vi "Write Packet.vi"(8 "error in (no error)":errorcluster, 9 "SessionMailbox in":refnum<queue>, 10 "Outgoing":T1, 11 "MQTT_Base in":refnum<class "MQTT_Base.lvclass">) -> (0 "error out":errorcluster, 3 "MQTT_Base out":refnum<class "MQTT_Base.lvclass">)   [LabVIEW 2013, in "MQTT Base.lvlib" / "MQTT_Base.lvclass"]
uses:
  MQTT_Base.lvclass
  Response -- cluster.ctl
  <vilib>/LabVIEW Open Source Project/MQTT Control Packets/Control Packets/ControlPacket/ControlPacket.lvclass
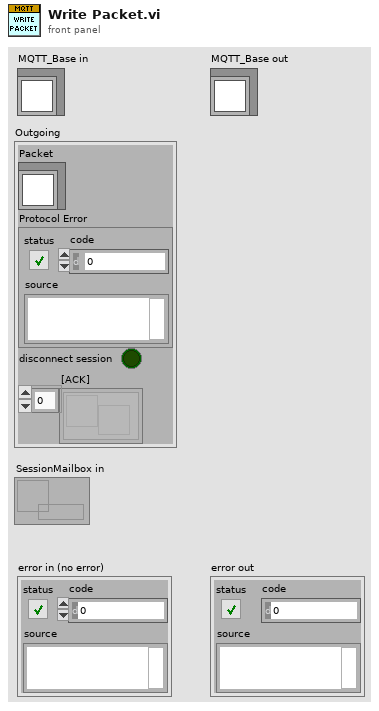
[diagram p1: front panel]
types:
  T1 = typedef "MQTT Base.lvlib/MQTT_Base.lvclass/Response -- cluster.ctl" = cluster{"Packet":refnum<class "ControlPacket.lvclass">, "Protocol Error":errorcluster, "disconnect session":bool, "[ACK]":refnum<notifier>[]}
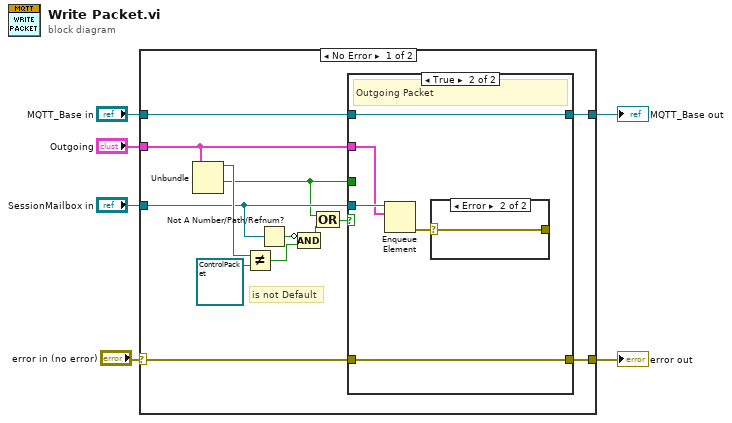
[diagram p0: block diagram]
diagram:
  n1 = case shown="No Error" "error in (no error)" {
    selector: "error in (no error)" -> [w8 w30]
    tunnel: "Outgoing" -> [w16 _]
    tunnel: "SessionMailbox in" -> [w15 _]
    tunnel: [w14 w30] -> w4
    tunnel: [w13 w29] -> w3
    tunnel: "MQTT_Base in" -> [w12 w29]
    frame No Error {
      # "is not Default"
      n2 = Unbundle(w16) -> ("Packet"=w17:refnum<class "ControlPacket.lvclass">, "disconnect session"=w7:bool)  [unwired: 2 out]
      n3 = Not Equal?(x=w17, y=refnum<class "ControlPacket.lvclass"> refnum ("ControlPacket.lvclass")) -> (x != y?=w11:bool)
      n4 = Not A Number/Path/Refnum?(number/path/refnum=w15) -> (NaN/Path/Refnum?=w10:bool)
      n5 = Compound Arithmetic op=AND(invert w10, w11) -> (w18:bool)
      n6 = Compound Arithmetic op=OR(w7, w18) -> (w19:bool)
      n7 = case shown="True" w19 {
        tunnel: w16 -> [_ w23]
        tunnel: w15 -> [_ w26]
        tunnel: w8 -> [w20 w24]
        tunnel: w12 -> [w21 w25]
        tunnel: [w21 w25] -> w13
        tunnel: [w20 w24] -> w14
        tunnel: w7 -> [_ _]
        frame False {
        }
        frame True {
          # "Outgoing Packet"
          n8 = Enqueue Element(queue=w26, element=w23) -> (error out=w22:errorcluster)  [unwired: 2 in, 2 out]
          n9 = case shown="Error" w22 {
            selector: w22 -> [w27 w28]
            tunnel: [w27 w28] -> _
            frame No Error {
            }
            frame Error {
            }
          }
        }
      }
    }
    frame Error {
      # "#Question: \nOn Server Error, should we try to close all sessions here\nor let the destroy method do that."
    }
  }
  "error out" <- w4
  "MQTT_Base out" <- w3
